vi "check_if_empty.vi"(8 "error in (no error)":errorcluster, 11 "ErrorController":refnum<class "ErrorController.lvclass">) -> (0 "error out":errorcluster, 2 "empty?":bool, 3 "ErrorController":refnum<class "ErrorController.lvclass">)   [LabVIEW 2010, in "ErrorController.lvclass"]
uses:
  ErrorController.lvclass
  ErrorController.lvclass/ErrorController.ctl
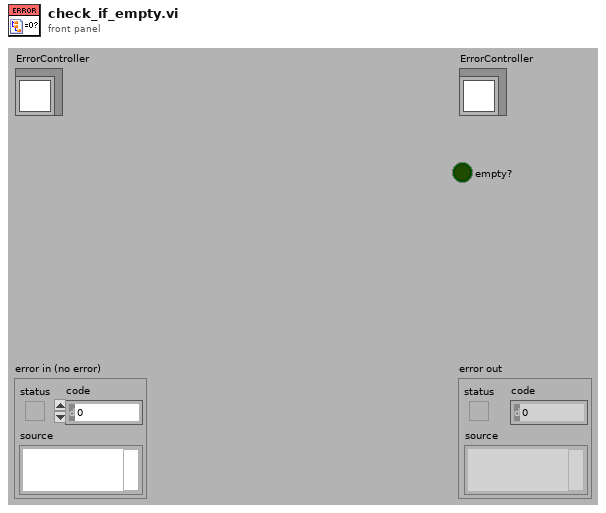
[diagram p1: front panel]
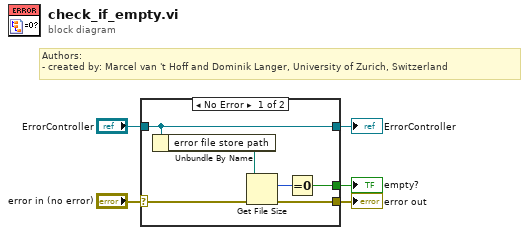
[diagram p0: block diagram]
diagram:
  # "Authors: \n- created by: Marcel van 't Hoff and Dominik Langer, University of Zurich, Switzerland"
  n1 = case shown="No Error" "error in (no error)" {
    selector: "error in (no error)" -> [w9 w13]
    tunnel: [w8 w13] -> w4
    tunnel: [w11 w12] -> w2
    tunnel: "ErrorController" -> [w11 w12]
    tunnel: [w6 _] -> w1
    frame No Error {
      n2 = Unbundle By Name(w11) -> ("error file store path"=w10:path)
      n3 = Get File Size(file=w10, error in=w9) -> (size (in bytes)=w7:i64, 0:w8:errorcluster)  [unwired: 1 out]
      n4 = Equal To 0?(x=w7) -> (x = 0?=w6:bool)
    }
    frame Error {
    }
  }
  "error out" <- w4
  "ErrorController" <- w2
  "empty?" <- w1
